vi "Single Sensor.vi"() -> ()   [LabVIEW 2019]
uses:
  <vilib>/Platform/TimedLoop/XDataNode/timing_clust.ctl
  <vilib>/Platform/TimedLoop/XDataNode/nitl_modes.ctl
  <vilib>/Platform/TimedLoop/XDataNode/wakeup.ctl
  <vilib>/myRIO/Instrument Drivers/Onboard IO/I2C/typedefs/I2C User Configuration.ctl
  <vilib>/myRIO/Instrument Drivers/Onboard IO/I2C/typedefs/I2C Transfer Rate.ctl
  <vilib>/myRIO/Instrument Drivers/Onboard IO/I2C/typedefs/I2C Reference.ctl
  <vilib>/myRIO/Common/Instrument Driver Framework/Utilities/typedefs/myRIO Generic Hardware Reference.ctl
  <vilib>/myRIO/Common/Instrument Driver Framework/Utilities/typedefs/Hardware Version Enum.ctl
  <vilib>/myRIO/Common/Instrument Driver Framework/Utilities/typedefs/myRIO v1.0 Reference.ctl
  <vilib>/myRIO/Common/Instrument Driver Framework/Utilities/typedefs/Generic FPGA Reference.ctl
  <vilib>/myRIO/Common/Instrument Driver Framework/myRIO v1.0/I2C/typedefs/I2C Channels Enum.ctl
  <vilib>/myRIO/Instrument Drivers/Onboard IO/I2C/typedefs/I2C Configuration.ctl
  <vilib>/userDefined/High Color/nirio_resource_hc.ctl
  <vilib>/myRIO/Common/Instrument Driver Framework/Utilities/vis/Is FPGA Ref Available.vi
  <vilib>/myRIO/Common/Instrument Driver Framework/myRIO v1.0/I2C/vis/myRIO v1.1 Open I2C.vi
  <vilib>/myRIO/Instrument Drivers/Onboard IO/I2C/vis/Configure.vi
  <vilib>/myRIO/Instrument Drivers/Onboard IO/I2C/vis/Write.vi
  <vilib>/myRIO/Instrument Drivers/Onboard IO/I2C/vis/Write Read.vi
  <vilib>/myRIO/Common/Instrument Driver Framework/Utilities/vis/Validate Channels.vi
  <vilib>/myRIO/Common/Instrument Driver Framework/myRIO v1.0/I2C/vis/myRIO v1.0 Reserve I2C.vi
  <vilib>/myRIO/Common/Instrument Driver Framework/myRIO v1.0/UART/vis/myRIO v1.0 Close UART.vi
  <vilib>/myRIO/Common/Instrument Driver Framework/myRIO v1.0/I2C/vis/myRIO v1.0 Build MUX Configuration I2C.vi
  <vilib>/myRIO/Common/Instrument Driver Framework/myRIO v1.0/Resource Manager/vis/myRIO v1.0 Reserve Channel List.vi
  <vilib>/myRIO/Common/Instrument Driver Framework/myRIO v1.0/Resource Manager/vis/myRIO v1.0 Create Configuration List.vi
  <vilib>/myRIO/Common/Instrument Driver Framework/myRIO v1.0/Resource Manager/vis/myRIO v1.0 Reserve Channel.vi
  <vilib>/myRIO/Common/Instrument Driver Framework/myRIO v1.0/Resource Manager/vis/myRIO v1.0 Unreserve Channel.vi
  <vilib>/myRIO/Common/Instrument Driver Framework/myRIO v1.0/Resource Manager/vis/myRIO v1.0 Build Mutex Name.vi
  <vilib>/Utility/VariantDataType/GetNumericInfo.vi
  <vilib>/Utility/error.llb/Error Cluster From Error Code.vi
  <vilib>/myRIO/Common/Instrument Driver Framework/myRIO v1.0/myRIO v1.1 Open.vi
  <vilib>/myRIO/Common/Instrument Driver Framework/Utilities/vis/IO Manager.vi
  <vilib>/myRIO/Common/Instrument Driver Framework/Utilities/vis/Configuration Manager.vi
  <vilib>/myRIO/Common/Instrument Driver Framework/myRIO v1.0/Resource Manager/vis/myRIO v1.0 Configure IO.vi
  <vilib>/myRIO/Common/Instrument Driver Framework/myRIO v1.0/myRIO v1.0 Close.vi
  <vilib>/myRIO/Common/Instrument Driver Framework/myRIO v1.0/I2C/vis/myRIO v1.0 Configure I2C.vi
  <vilib>/myRIO/Common/Instrument Driver Framework/myRIO v1.0/I2C/vis/myRIO v1.0 Write I2C.vi
  <vilib>/myRIO/Common/Instrument Driver Framework/myRIO v1.0/I2C/vis/myRIO v1.0 Read I2C.vi
  <vilib>/myRIO/Common/Instrument Driver Framework/Utilities/vis/FPGA Ref Manager.vi
  <vilib>/myRIO/Common/Instrument Driver Framework/myRIO v1.0/myRIO v1.0 Reset FPGA.vi
  <vilib>/myRIO/Common/Instrument Driver Framework/myRIO v1.0/IRQ/vis/myRIO v1.0 IRQ Info FGV.vi
  <vilib>/myRIO/Common/Instrument Driver Framework/myRIO v1.0/IRQ/vis/myRIO v1.0 Timer IRQ Info FGV.vi
  <vilib>/myRIO/Common/Instrument Driver Framework/myRIO v1.0/IRQ/vis/myRIO v1.0 ISR Agent.vi
  <vilib>/myRIO/Instrument Drivers/Utilities/vis/Reset Index.vi
  <vilib>/myRIO/Common/Instrument Driver Framework/myRIO v1.0/Resource Manager/vis/myRIO v1.0 Block Write Resource Manager.vi
  <vilib>/platform/TimedLoop/XDataNode/XDataNode.xnode
  <vilib>/myRIO/Express VI/Onboard IO/I2C/I2C Express VI.xnode
  <vilib>/myRIO/Instrument Drivers/Onboard IO/I2C/vis/myRIO I2C Open.xnode
  <vilib>/myRIO/Instrument Drivers/Utilities/Utilities.lvlib
  <vilib>/Platform/TimedLoop/XDataNode/XDNodeRunTimeDep.lvlib
  <vilib>/myRIO/Instrument Drivers/Onboard IO/I2C/I2C.lvlib
panel:
  out "Magnetic field [G]":cluster{dbl, dbl, dbl}(graph) caption="Waveform Chart"
  out "Z_mag":dbl
  out "Y_mag":dbl
  out "X_mag":dbl
  out "Magnetic field [LSb]":cluster{i16, i16, i16}(graph) caption="Waveform Chart"
  out "Z":i16
  out "Y":i16
  out "X":i16
  out "DATA":u8[](array[numeric]) format="%02x"
  in  "[ESC]":bool
  # "Compass demo"
  # "DATA_X_H"
  # "DATA_X_L"
  # "DATA_Z_H"
  # "DATA_Z_L"
  # "DATA_Y_H"
  # "DATA_Y_L"
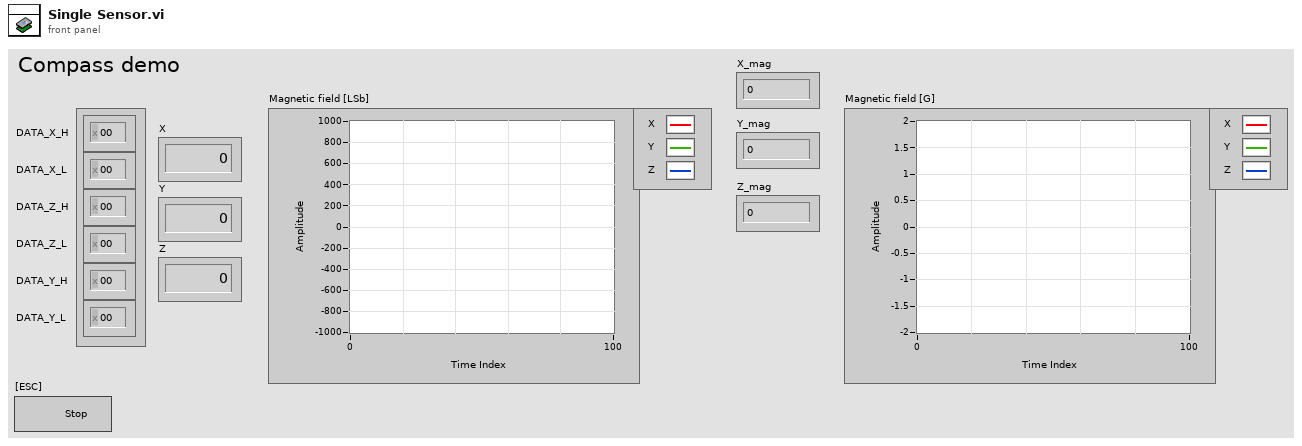
[diagram p1: front panel]
types:
  T1 = typedef "XDNodeRunTimeDep.lvlib/timing_clust.ctl" = cluster{"Expected End [f-1]":u64, "Actual End [f-1]":u64, "Finished Late? [f-1]":bool, "Expected End [i-1]":u64, "Actual End [i-1]":u64, "Finished Late? [i-1]":bool, "Expected Start [i]":u64, "Actual Start [i]":u64, "Expected Start [f]":u64, "Actual Start [f]":u64, "Source Name":string, "Structure Name":string, "Period":i64, "Deadline":i64, "Offset":i64, "Start":i64, "Priority":i32, "Timeout":i32, "Mode":T2, "Wakeup Reason":T3, "Error":errorcluster, "Source Type":string, "Secondary Source Type":string, "Global End Time":u64, "Global Start Time":u64, "Frame Duration":u64, "Iteration Duration":u64, "Assigned CPU":i32, "I/O Scan Engine Mode":u32}
  T2 = typedef "XDNodeRunTimeDep.lvlib/nitl_modes.ctl" = enum32{"No Change", "Process missed periods, maintain original phase", "Discard missed periods, maintain original phase", "Process missed periods, ignore original phase", "Discard missed periods, ignore original phase"}
  T3 = typedef "XDNodeRunTimeDep.lvlib/wakeup.ctl" = enum32{"Normal", "Aborted", "Asynchronous wakeup", "Timing source error", "Timed loop error", "Timeout"}
  T4 = typedef "I2C.lvlib/I2C Reference.ctl" = cluster{"myRIO Reference":T5, "I2C Channels Enum":T9, "I2C Configuration":T10}
  T5 = typedef "myRIO Generic Hardware Reference.ctl" = cluster{"myRIO Model":T6, "myRIO Hardware Reference":T7}
  T6 = typedef "Hardware Version Enum.ctl" = enum16{"Unknown", "myRIO-1900", "myRIO-1950", "roboRIO", "NI ELVIS RIO CM", "ELVIS III"}
  T7 = typedef "myRIO v1.0 Reference.ctl" = cluster{"Generic FPGA Reference":T8, "Allow multiple opens":bool}
  T8 = typedef "Generic FPGA Reference.ctl" = refnum<k20>
  T9 = typedef "I2C Channels Enum.ctl" = enum16{"Not Connected", "A/I2C", "B/I2C", "I2C/I2C"}
  T10 = typedef "I2C.lvlib/I2C Configuration.ctl" = cluster{"I2C Transfer Rate":T11}
  T11 = typedef "I2C.lvlib/I2C Transfer Rate.ctl" = enum16{"Standard mode (100 kbps)", "Fast mode (400 kbps)"}
  T12 = typedef "I2C.lvlib/I2C User Configuration.ctl" = cluster{"I2C Transfer Rate":T11}
  T13 = typedef "nirio_resource_hc.ctl" = tag
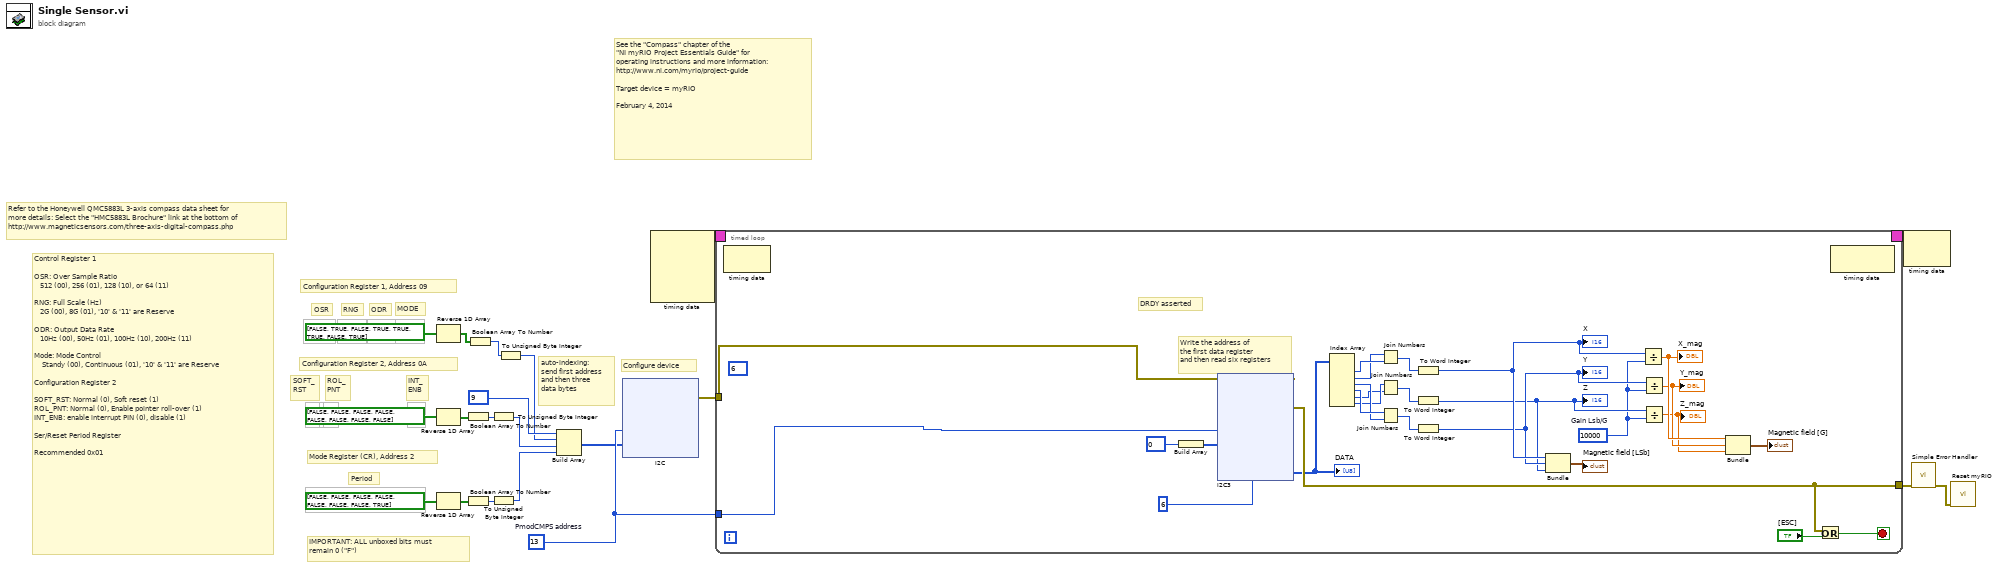
[diagram p0: block diagram]
diagram:
  w4 = u8 13  # PmodCMPS address
  # "INT_\nENB"
  # "ROL_\nPNT"
  # "ODR"
  # "See the \"Compass\" chapter of the\n\"NI myRIO Project Essentials Guide\" for\noperating instructions and more information: \nhttp://www.ni.com/myrio/project-guide\n\nTarget device = myRIO\n\nFebruary 4, 2014"
  # "Refer to the Honeywell QMC5883L 3-axis compass data sheet for \nmore details: Select the \"HMC5883L Brochure\" link at the bottom of\nhttp://www.magneticsensors.com/three-axis-digital-compass.php"
  # "auto-indexing:\nsend first address\nand then three\ndata bytes"
  # "Control Register 1\n\nOSR: Over Sample Ratio \n   512 (00), 256 (01), 128 (10), or 64 (11)\n\nRNG: Full Scale (Hz)\n   2G (00), 8G (01), '10' & '11' are Reserve\n\nODR: Output Data Rate\n   10Hz (00), 50Hz (01), 100Hz (10), 200Hz (11)\n\nMode: Mode Control\n    Standy (00), Continuous (01), '10' & '11' are Reserve     \n\nConfiguration Register 2\n\nSOFT_RST: Normal (0), Soft reset (1)\nROL_PNT: Normal (0), Enable pointer roll-over (1)\nINT_ENB: enable interrupt PIN (0), disable (1)\n\nSer/Reset Period Register\n\nRecommended 0x01"
  # "IMPORTANT: ALL unboxed bits must\nremain 0 (\"F\")"
  # "Configure device"
  # "Period"
  # "Mode Register (CR), Address 2"
  # "Configuration Register 2, Address 0A"
  # "SOFT_\nRST"
  # "Configuration Register 1, Address 09"
  # "MODE"
  # "RNG"
  # "OSR"
  n1 = Reverse 1D Array(array=bool[] [FALSE, TRUE, FALSE, TRUE, TRUE, TRUE, FALSE, TRUE]) -> (reversed array=w15:bool[])
  n2 = Reverse 1D Array(array=bool[] [FALSE, FALSE, FALSE, FALSE, FALSE, FALSE, FALSE, FALSE]) -> (reversed array=w14:bool[])
  n3 = Reverse 1D Array(array=bool[] [FALSE, FALSE, FALSE, FALSE, FALSE, FALSE, FALSE, TRUE]) -> (reversed array=w12:bool[])
  n4 = Boolean Array To Number(Boolean array=w14) -> (number=w8:u32)
  n5 = Boolean Array To Number(Boolean array=w12) -> (number=w7:u32)
  n6 = Boolean Array To Number(Boolean array=w15) -> (number=w9:u32)
  n7 = To Unsigned Byte Integer(number=w8) -> (unsigned 8bit integer=w2:u8)
  n8 = To Unsigned Byte Integer(number=w7) -> (unsigned 8bit integer=w1:u8)
  n9 = To Unsigned Byte Integer(number=w9) -> (unsigned 8bit integer=w6:u8)
  n10 = Build Array "Build Array"(u8 9 ("address"), w6, w2, w1) -> (w3:u8[])
  n11 = xnode "I2C"("Slave Address (7-bit)"=w4, "Bytes to Write"=w3) -> ("error out"=w5:errorcluster)  [unwired: 1 in]
  n12 = node-c288() -> (w18:T1)  [unwired: 4 in]
  n13 = timed-loop {
    tunnel: [w45] -> w19
    tunnel: w5 -> [w22]
    tunnel: w4 -> [w21]
    timing: w18 -> [_]
    timing-out: [_] -> w17
    stop <- w47 stop-if-true
    w33 = i16 10000  # Gain Lsb/G
    (unwired) u8 6
    # "DRDY asserted"
    # "Write the address of\nthe first data register\nand then read six registers"
    n14 = node-c288() -> ()  [unwired: 1 in, 1 out]
    n15 = Build Array(u8 0) -> (w38:u8[])
    n16 = xnode "I2C3"("Slave Address (7-bit)"=w21, "Bytes to Write"=w38, "Byte Count"=u32 6, "error in (no error)"=w22) -> ("Bytes Read"=w41:u8[], "error out"=w45:errorcluster)
    "DATA" <- w41
    n17 = Index Array "Index Array"(array=w41) -> (element #1=w28:u8, element #2=w27:u8, element #3=w25:u8, element #4=w26:u8, element #5=w23:u8, element #6=w24:u8)  [unwired: 6 in]
    n18 = Join Numbers(hi=w27, lo=w28) -> ((hi.lo)=w44:u16)
    n19 = Join Numbers(hi=w24, lo=w23) -> ((hi.lo)=w43:u16)
    n20 = Join Numbers(hi=w26, lo=w25) -> ((hi.lo)=w42:u16)
    n21 = To Word Integer(number=w44) -> (16bit integer=w36:i16)
    "X" <- w36
    n22 = To Word Integer(number=w43) -> (16bit integer=w34:i16)
    "Z" <- w34
    n23 = To Word Integer(number=w42) -> (16bit integer=w35:i16)
    "Y" <- w35
    n24 = Bundle(w36, w35, w34) -> (→"Magnetic field [LSb]":cluster{i16, i16, i16})  [unwired: 1 in]
    n25 = Divide(x=w36, y=w33) -> (x/y=w32:dbl)
    "X_mag" <- w32
    n26 = Divide(x=w35, y=w33) -> (x/y=w31:dbl)
    "Y_mag" <- w31
    n27 = Divide(x=w34, y=w33) -> (x/y=w30:dbl)
    "Z_mag" <- w30
    n28 = Bundle(w32, w31, w30) -> (→"Magnetic field [G]":cluster{dbl, dbl, dbl})  [unwired: 1 in]
    n29 = Or(x=w45, y="[ESC]") -> (x .or. y?=w47:bool)
    n30 = node-c288() -> ()  [unwired: 1 in, 1 out]
  }
  n31 = node-c288(w17) -> ()  [unwired: 1 out]
  n32 = call <vilib>:"Simple Error Handler.vi"("error in (no error)"=w19) -> ("error out"=w20:errorcluster)  [unwired: 4 in, 4 out]
  n33 = call <vilib>:"Reset myRIO.vi"("error in (no error)"=w20) -> ()  [unwired: 10 in, 1 out]
